vi "U3 DAC0 and AIN2 Diff.vi"() -> ()   [LabVIEW 2021]
panel:
  in  "Iteration Interval (ms)":i32=100
  in  "stop":bool
  out "AIN2":dbl format="%.6f"
  in  "DAC0":dbl step=0.1 format="%.4f"
  out "Error Message":string
  out "error out":errorcluster
  # "Outputs DAC0 and aquires AIN2.  AIN2 is measured differentially compared\nto Vref.  The special negative channel 32 is used, such that Vref is added\nto the reading, resulting in a single-ended range on the positive channel of\nabout 0-3.6 volts."
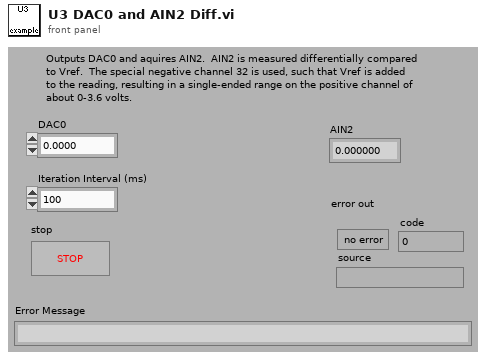
[diagram p1: front panel]
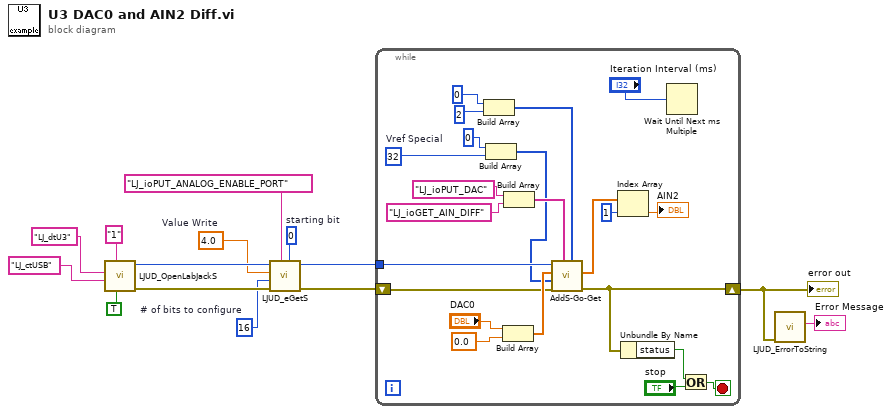
[diagram p0: block diagram]
diagram:
  w3 = 16  # # of bits to configure
  w5 = 0  # starting bit
  w6 = 4.0  # Value Write
  n1 = call "LJUD_OpenLabJackS.vi"("FirstFound"=TRUE, "Address"="1", "ConnectionType"="LJ_ctUSB", "DeviceType"="LJ_dtU3") -> ("error out"=w8:errorcluster, "Handle"=w9:i32)  [unwired: 5 in, 1 out]
  n2 = call "LJUD_eGetS.vi"("Channel"=w5, "IOType"="LJ_ioPUT_ANALOG_ENABLE_PORT", "error in"=w8, "x1"=w3, "Value Write"=w6, "Handle In"=w9) -> ("error out"=w2:errorcluster, "Handle Out"=w7:i32)  [unwired: 3 in, 1 out]
  n3 = while {
    shift-left: w2 -> [w23]
    shift-right: [w20] -> w1
    tunnel: w7 -> [w31]
    stop <- w22 stop-if-true
    w16 = 32  # Vref Special
    n4 = Build Array(0, 2) -> (w35:i32[])
    n5 = Build Array(0, w16) -> (w15:i32[])
    n6 = Build Array("DAC0", 0.0 ("Input Element")) -> (w34:dbl[])
    n7 = Build Array("LJ_ioPUT_DAC" ("IOType"), "LJ_ioGET_AIN_DIFF" ("IOType")) -> (w36:string[])
    n8 = call "AddS-Go-Get.vi"("Channels"=w35, "IOTypes"=w36, "error in"=w23, "x1"=w15, "Values Write"=w34, "Handle In"=w31) -> ("error out"=w20:errorcluster, "Values Read"=w25:dbl[])  [unwired: 3 in, 1 out]
    n9 = Index Array(array=w25, index=1 ("Index")) -> (element=→"AIN2":dbl)
    n10 = Unbundle By Name(w20) -> ("status"=w19:bool)
    n11 = Wait Until Next ms Multiple(millisecond multiple="Iteration Interval (ms)") -> ()  [unwired: 1 out]
    n12 = Or(x=w19, y="stop") -> (x .or. y?=w22:bool)
  }
  "error out" <- w1
  n13 = call "LJUD_ErrorToString.vi"("error in"=w1) -> ("String"=→"Error Message":string)  [unwired: 10 in]
